vi "Set_parameter.vi"(6 "Delete last CMD":bool, 8 "error in (no error)":errorcluster, 9 "value":dbl, 10 "parameter":string, 11 "Dali_usb_tridonics in":refnum<class "Dali_usb_tridonics.lvclass">) -> (0 "error out":errorcluster, 3 "Dali_usb_tridonics out":refnum<class "Dali_usb_tridonics.lvclass">)   [LabVIEW 2014, in "Driver_interaction.lvlib" / "Dali_usb_tridonics.lvclass"]
uses:
  Dali_usb_tridonics.lvclass
  Dali_usb_tridonics.lvclass/Dali_usb_tridonics.ctl
  Vendor/Controls/Addressing_type.ctl
  _Driver_interaction/_Driver_interaction.lvclass
  Vendor/Dali_usb.lvlib
panel:
  out "Responses":string[](array[string])
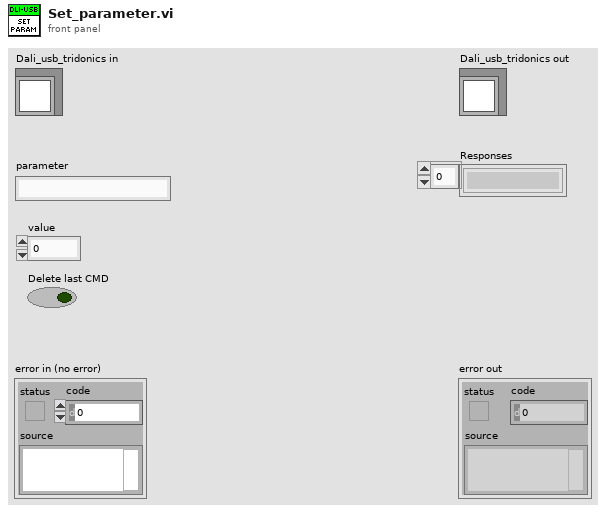
[diagram p1: front panel]
types:
  T1 = typedef "Dali_usb.lvlib/Addressing_type.ctl" = string
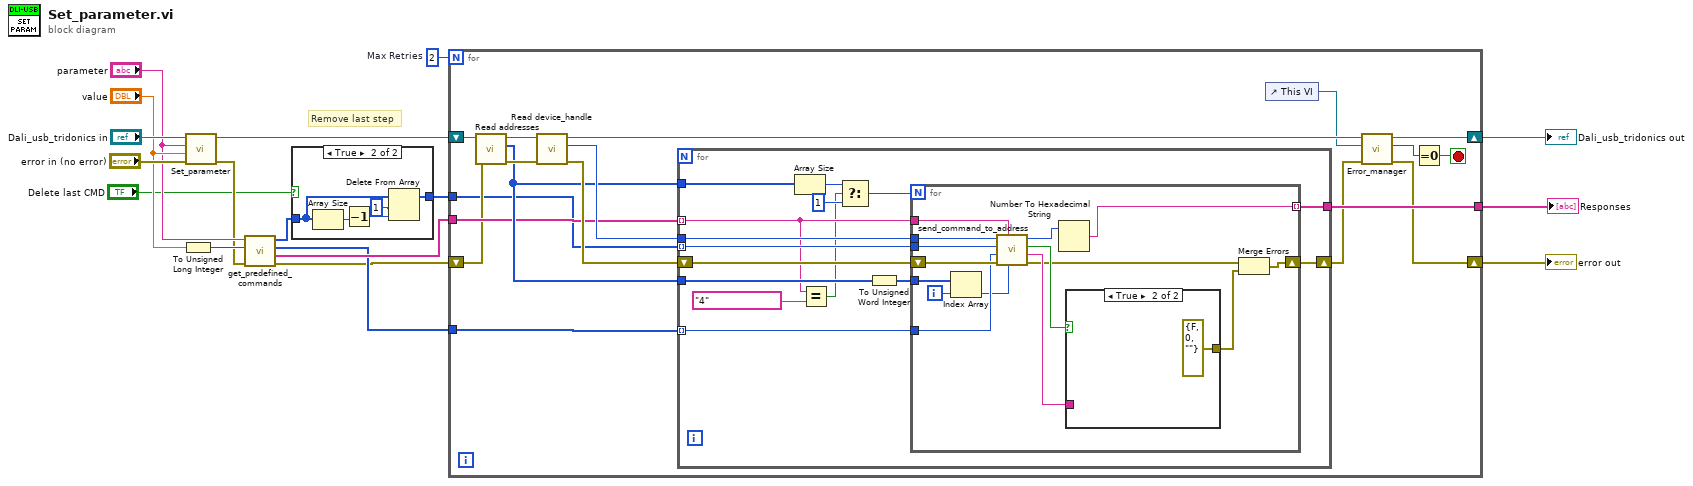
[diagram p0: block diagram]
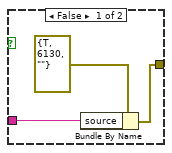
[diagram p2: hidden frame]
diagram:
  w2 = 2  # Max Retries
  # "Remove last step"
  n1 = To Unsigned Long Integer(number="value") -> (unsigned 32bit integer=w8:u32)
  n2 = call-parent "Set_parameter.vi"("error in (no error)"="error in (no error)", "value"="value", "parameter"="parameter", "_Driver_interaction in"="Dali_usb_tridonics in") -> ("error out"=w7:errorcluster, "_Driver_interaction out"=w14:refnum<class "Dali_usb_tridonics.lvclass">)  [unwired: 6 in]
  n3 = call "get_predefined_commands.vi"("error in (no error)"=w7, "value_to_set"=w8, "Predefined_routines"="parameter") -> ("error out"=w6:errorcluster, "addressings"=w10:T1[], "data"=w9:u32[], "commands"=w5:u32[])  [unwired: 5 in]
  n4 = case shown="True" "Delete last CMD" {
    tunnel: w5 -> [w18 w22]
    tunnel: [w18 w19] -> w4
    frame False {
    }
    frame True {
      n5 = Array Size(array=w22) -> (size(s)=w21:i32)
      n6 = Decrement(x=w21) -> (x-1=w20:i32)
      n7 = Delete From Array(array=w22, length=1, index=w20) -> (array with subset deleted=w19:u32[])  [unwired: 1 out]
    }
  }
  n8 = for {
    N: w2 -> [_]
    tunnel: [w35] -> w11
    tunnel: w10 -> [w34]
    tunnel: w9 -> [w33]
    tunnel: w4 -> [w31]
    shift-right: [w27] -> w13
    shift-left: w14 -> [w39]
    shift-right: [w29] -> w1
    shift-left: w6 -> [w32]
    stop <- w25 stop-if-true
    n9 = call "Read addresses.vi"("error in (no error)"=w32, "Dali_usb_tridonics in"=w39) -> ("error out"=w40:errorcluster, "addresses"=w36:i32[], "Dali_usb_tridonics out"=w41:refnum<class "Dali_usb_tridonics.lvclass">)  [unwired: 7 in]
    n10 = call "Read device_handle.vi"("error in (no error)"=w40, "Dali_usb_tridonics in"=w41) -> ("error out"=w38:errorcluster, "device_handle"=w37:i32, "Dali_usb_tridonics out"=w28:refnum<class "Dali_usb_tridonics.lvclass">)  [unwired: 7 in]
    n11 = for {
      tunnel: w31 -> [w56] mode=indexing
      tunnel: w37 -> [w55]
      tunnel: w36 -> [w53]
      tunnel: [w51] -> w35
      shift-right: [w50] -> w30
      shift-left: w38 -> [w54]
      tunnel: w34 -> [w45] mode=indexing
      tunnel: w36 -> [w49]
      tunnel: w33 -> [w43] mode=indexing
      n12 = Array Size(array=w49) -> (size(s)=w48:i32)
      n13 = Equal?(x=w45, y=T1 "4" ("Addresing")) -> (x = y?=w44:bool)
      n14 = Select(t=w48, s=w44, f=1) -> (s? t:f=w47:i32)
      n15 = To Unsigned Word Integer(number=w53) -> (unsigned 16bit integer=w52:u16[])
      n16 = for {
        N: w47 -> [_]
        tunnel: w52 -> [w59]
        tunnel: w56 -> [w70]
        tunnel: w55 -> [w71]
        shift-right: [w62] -> w50
        shift-left: w54 -> [w69]
        tunnel: [w65] -> w51 mode=indexing
        tunnel: w45 -> [w61]
        tunnel: w43 -> [w58]
        i -> [w60]
        n17 = Index Array(array=w59, index=w60) -> (element=w57:u16)
        n18 = call "send_command_to_address.vi"("address_group"=w57, "addressing_type"=w61, "error in (no error)"=w69, "command_data"=w58, "command"=w70, "device_handle"=w71) -> ("error out"=w64:errorcluster, "failstring"=w67:string, "ok"=w68:bool, "response_command"=w66:i32)  [unwired: 2 in]
        n19 = Number To Hexadecimal String(2:w66) -> (0:w65:string)  [unwired: 1 in]
        n20 = case shown="True" w68 {
          tunnel: w67 -> [w73 _]
          tunnel: [w72 errorcluster {"status"=FALSE, "code"=0, "source"=""} ("error out")] -> w63
          frame False {
            n21 = Bundle By Name(cluster=errorcluster {"status"=TRUE, "code"=6130, "source"=""} ("error out"), "source"=w73) -> (w72:errorcluster)
          }
          frame True {
          }
        }
        n22 = Merge Errors(w64, w63) -> (w62:errorcluster)
      }
    }
    n23 = control-ref of="This VI"() -> (w24:refnum<vi>)
    n24 = call-dynamic "Error_manager.vi"("error in (no error)"=w30, "Caller VI"=w24, "Dali_usb_tridonics in"=w28) -> ("error out"=w29:errorcluster, "code"=w26:i32, "Dali_usb_tridonics out"=w27:refnum<class "Dali_usb_tridonics.lvclass">)  [unwired: 4 in, 2 out]
    n25 = Equal To 0?(x=w26) -> (x = 0?=w25:bool)
  }
  "error out" <- w1
  "Dali_usb_tridonics out" <- w13
  "Responses" <- w11
